vi "ContinousToDiscrete.vi"(8 "R":T1, 9 "Q":T1, 10 "B":T1=[[0.0], [1.0]], 11 "A":T1=[[0.0, 1.0], [0.0, -1.0]]) -> (2 "B_d":T1=[[0.00019867330675530227], [0.0198013266932447]], 3 "A_d":T1=[[1.0, 0.0198013266932447], [0.0, 0.9801986733067554]])   [LabVIEW 2017]
uses:
  <vilib>/Analysis/Matrix/Datatypes/RealMatrix.ctl
  <vilib>/Analysis/7linalg.llb/Real Matrix Exp.vi
  <vilib>/Analysis/Matrix/Numeric/Multiply/Multiply - RM,R.vi
  <vilib>/Analysis/Matrix/NI_Matrix.lvlib
  <vilib>/Analysis/NI_AALBase.lvlib
panel:
  in  "dt":dbl=0.01
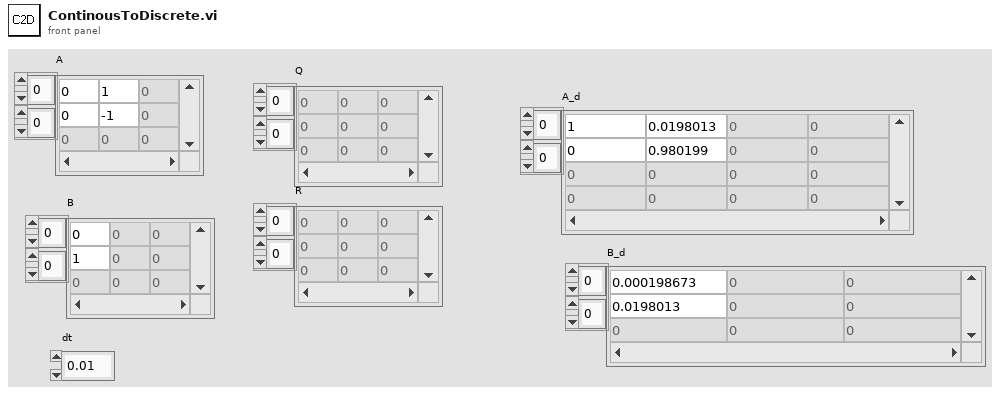
[diagram p1: front panel]
types:
  T1 = typedef "NI_Matrix.lvlib/RealMatrix.ctl" = dbl[][]
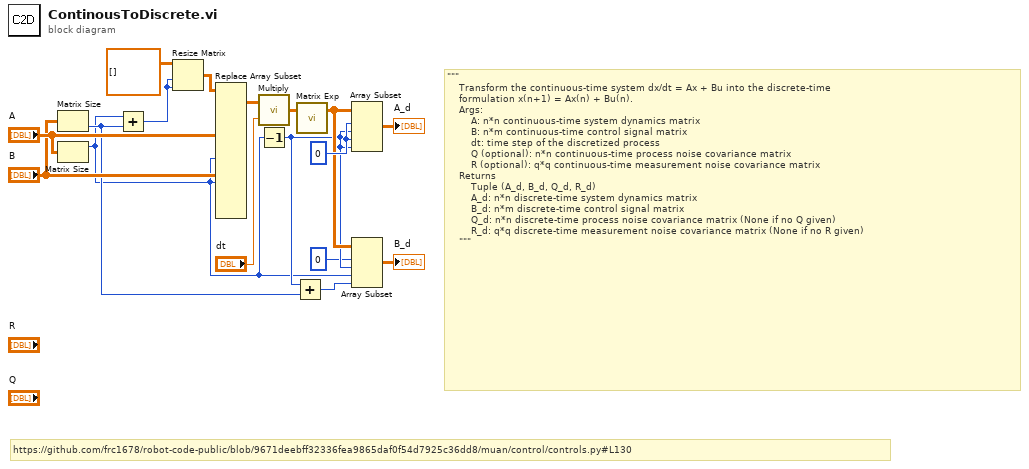
[diagram p0: block diagram]
diagram:
  w8 = 0 ("row 1")
  # "\"\"\"\n    Transform the continuous-time system dx/dt = Ax + Bu into the discrete-time\n    formulation x(n+1) = Ax(n) + Bu(n).\n    Args:\n        A: n*n continuous-time system dynamics matrix\n        B: n*m continuous-time control signal matrix\n        dt: time step of the discretized process\n        Q (optional): n*n continuous-time process noise covariance matrix\n        R (optional): q*q continuous-time measurement noise covariance matrix\n    Returns\n        Tuple (A_d, B_d, Q_d, R_d)\n        A_d: n*n discrete-time system dynamics matrix\n        B_d: n*m discrete-time control signal matrix\n        Q_d: n*n discrete-time process noise covariance matrix (None if no Q given)\n        R_d: q*q discrete-time measurement noise covariance matrix (None if no R given)\n    \"\"\""
  # "https://github.com/frc1678/robot-code-public/blob/9671deebff32336fea9865daf0f54d7925c36dd8/muan/control/controls.py#L130"
  n1 = Matrix Size(0:"B") -> (2:w3:i32)  [unwired: 1 out]
  n2 = Matrix Size(0:"A") -> (1:w1:i32)  [unwired: 1 out]
  n3 = Add(x=w1, y=w3) -> (x+y=w17:i32)
  n4 = Resize Matrix(1:w17, 2:w17, 4:T1 [] ("matrix")) -> (0:w15:T1)
  n5 = Replace Array Subset(array=w15, new element #1="A", new element #2="B", index (dim 2) #2=w1, index (dim 0) #3=w1) -> (w12:T1)  [unwired: 11 in]
  n6 = call-poly <vilib>:"Multiply.vi"("Real Scalar c"="dt", "Real Matrix A"=w12) -> ("A * c"=w10:T1)
  n7 = Decrement(x=w1) -> (x-1=w4:i32)
  n8 = Add(x=w4, y=w3) -> (x+y=w5:i32)
  n9 = call-poly <vilib>:"Matrix Exp.vi"("Input Matrix"=w10) -> ("Matrix Exp"=w7:T1)  [unwired: 1 in, 1 out]
  n10 = Array Subset(array=w7, index (row)=w8, length (row)=w4, index (col)=w8, length (col)=w4) -> (→"A_d":T1)
  n11 = Array Subset(array=w7, index (row)=0 ("row 1"), length (row)=w4, index (col)=w1, length (col)=w5) -> (→"B_d":T1)
